vi "SetCurrentRange.vi"(2 "string":string, 3 "error out 2":errorcluster, 4 "reference out 2":refnum<visa-resource-name>) -> (0 "error out":errorcluster, 1 "reference out":refnum<visa-resource-name>)   [LabVIEW 2009]
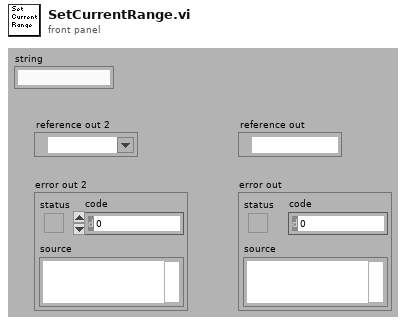
[diagram p1: front panel]
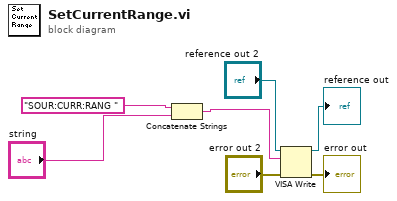
[diagram p0: block diagram]
diagram:
  n1 = Concatenate Strings("SOUR:CURR:RANG " ("write buffer"), "string") -> (w2:string)
  n2 = VISA Write(VISA resource name="reference out 2", write buffer=w2, error in (no error)="error out 2") -> (VISA resource name out=→"reference out":refnum<visa-resource-name>, error out=→"error out":errorcluster)  [unwired: 1 out]
